vi "SetVariant(Attr).vi"(8 "error in (no error)":errorcluster, 10 "[Attributes]":variant, 11 "SMO in":refnum<class "SMO.lvclass">) -> (0 "error out":errorcluster, 3 "SMO out":refnum<class "SMO.lvclass">)   [LabVIEW 2013, in "SMO.lvclass"]
uses:
  SMO.lvclass
  SMO.lvclass/SMO.ctl
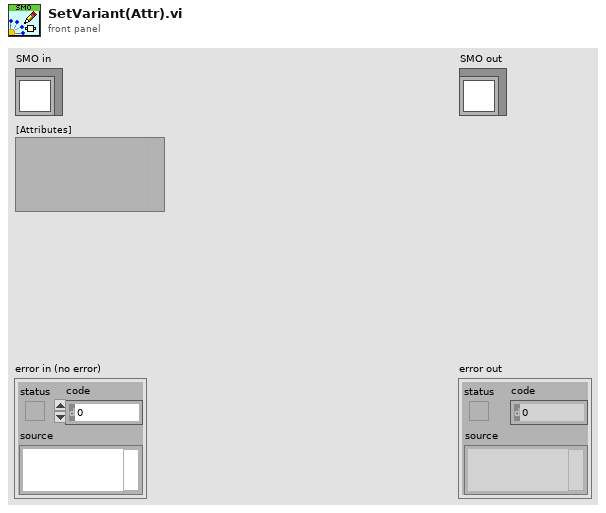
[diagram p1: front panel]
types:
  T1 = typedef "SMO.lvclass/PrivateData--Ref.ctl" = refnum<data-value>
  T2 = typedef "SMO.lvclass/PrivateData--Cluster.ctl" = cluster{"Parent Call":T3, "Registered Processes":T4[], "Sync Notifier":refnum<notifier>, "Process Error Notifier":refnum<notifier>, "Protected Events":T5, "Public Events":T6, "SMO State":T7, "[Dependencies]":T8[], "[Attributes]":variant, "Launcher Close":refnum<notifier>, "Caller Watchdog":refnum<queue>, "Accessibility":T9, "NbStaticDependencies":u32}
  T3 = typedef "SMO.lvclass/Parent Call--Enum.ctl" = enum16{"Allows parent to run", "Does not request parent to run"}
  T4 = typedef "SMO.lvclass/RegisteredProcessData--Cluster.ctl" = cluster{"Name":string, "Static VI Ref":refnum<vi>, "Running":bool, "NotifierRef":u32}
  T5 = typedef "SMO.lvclass/Protected Events.ctl" = cluster{"StopProcesses":refnum<user-event>, "AbortProcesses":refnum<user-event>, "Config Changed":refnum<user-event>, "Dependency":refnum<user-event>}
  T6 = typedef "SMO.lvclass/Public Events.ctl" = cluster{"Error":refnum<user-event>, "State":refnum<user-event>, "Reserve State":refnum<user-event>}
  T7 = typedef "SMO.lvclass/SMOState --Enum.ctl" = enum16{"unknown", "Created", "Started", "Stopped"}
  T8 = typedef "SMO.lvclass/SMO Dependency--Cluster.ctl" = cluster{"Dependency":refnum<class "SMO.lvclass">, "Level":string}
  T9 = typedef "SMO.lvclass/Accessibility--Cluster.ctl" = cluster{"Lock Key":string, "Reserve State":T10}
  T10 = typedef "SMO.lvclass/Reserve State--Enum.ctl" = enum16{"Unreserved", "Reserved", "Self-locked"}
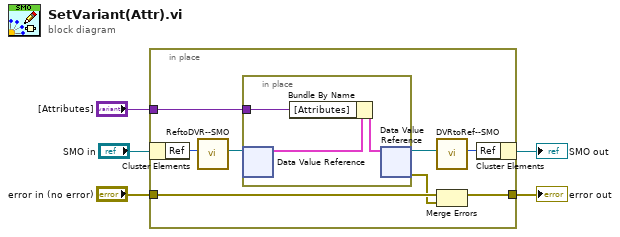
[diagram p0: block diagram]
diagram:
  n1 = in-place {
    in-place-border: "error in (no error)" -> [w9]
    in-place-border: [w7] -> w2
    in-place-border: "[Attributes]" -> [w6]
    n2 = in-place-cluster #1("SMO in") -> ("Ref"=w13:u32)
    n3 = call "ReftoDVR--SMO.vi"("Ref"=w13) -> ("Ref"=w12:T1)  [unwired: 10 in]
    n4 = in-place {
      in-place-border: w6 -> [w14]
      n5 = in-place-dvr #2(w12) -> (w16:T2)  [unwired: 1 out]
      n6 = Bundle By Name(cluster=w16, "[Attributes]"=w14) -> (w15:T2)
      n7 = in-place-dvr #2(w15) -> (w11:T1, w8:errorcluster)
    }
    n8 = call "DVRtoRef--SMO.vi"("Ref"=w11) -> ("Ref"=w10:u32)  [unwired: 10 in]
    n9 = Merge Errors(w9, w8) -> (w7:errorcluster)
    n10 = in-place-cluster #1("Ref"=w10) -> (→"SMO out":refnum<class "SMO.lvclass">)
  }
  "error out" <- w2
